vi "Increment Matrix.vi"(10 "Value to add":u8, 11 "Data Matrix In":u8[][](array[numeric])) -> (3 "Data Matrix Out":u8[][](array[numeric]))   [LabVIEW 2019, in "Day 15.lvlib"]
uses:
  Day 15.lvlib
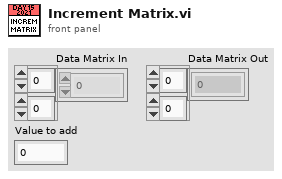
[diagram p1: front panel]
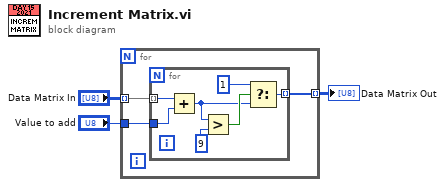
[diagram p0: block diagram]
diagram:
  n1 = for {
    tunnel: "Data Matrix In" -> [w6] mode=indexing
    tunnel: "Value to add" -> [w5]
    tunnel: [w4] -> w1 mode=indexing
    n2 = for {
      tunnel: w6 -> [w13] mode=indexing
      tunnel: w5 -> [w11]
      tunnel: [w7] -> w4 mode=indexing
      n3 = Add(x=w13, y=w11) -> (x+y=w8:u8)
      n4 = Greater?(x=w8, y=u8 9) -> (0:w10:bool)
      n5 = Select(t=u8 1 ("y"), s=w10, f=w8) -> (s? t:f=w7:u8)
    }
  }
  "Data Matrix Out" <- w1
